vi "Trama_RMC(SubVI).vi"(0 "TRAMA":string) -> (1 "Fecha":T3, 2 "output cluster":T1, 3 "Hora":T2, 4 "Cluster":T4)   [LabVIEW 2020]
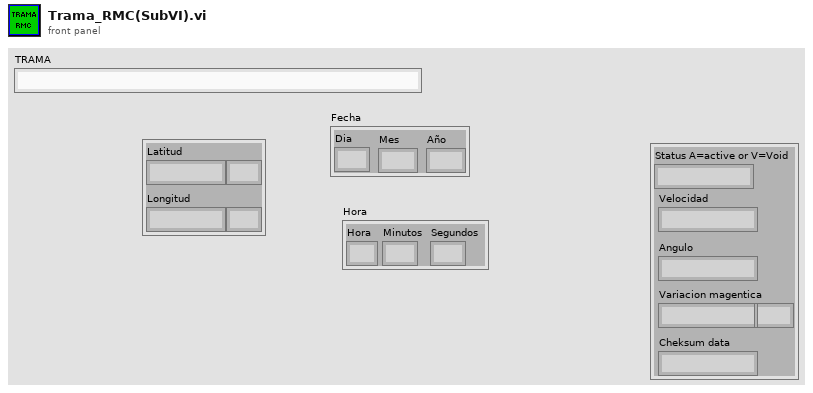
[diagram p1: front panel]
types:
  T1 = cluster{"Latitud":string, string, "Longitud":string, string}
  T2 = cluster{"Hora":string, "Segundos":string, "Minutos":string}
  T3 = cluster{"Dia":string, "Mes":string, "Año":string}
  T4 = cluster{"Status A=active or V=Void":string, "Velocidad":string, "Angulo":string, "Variacion magentica":string, string, "Cheksum data":string}
  T5 = cluster{string, string, string, string, string, string}
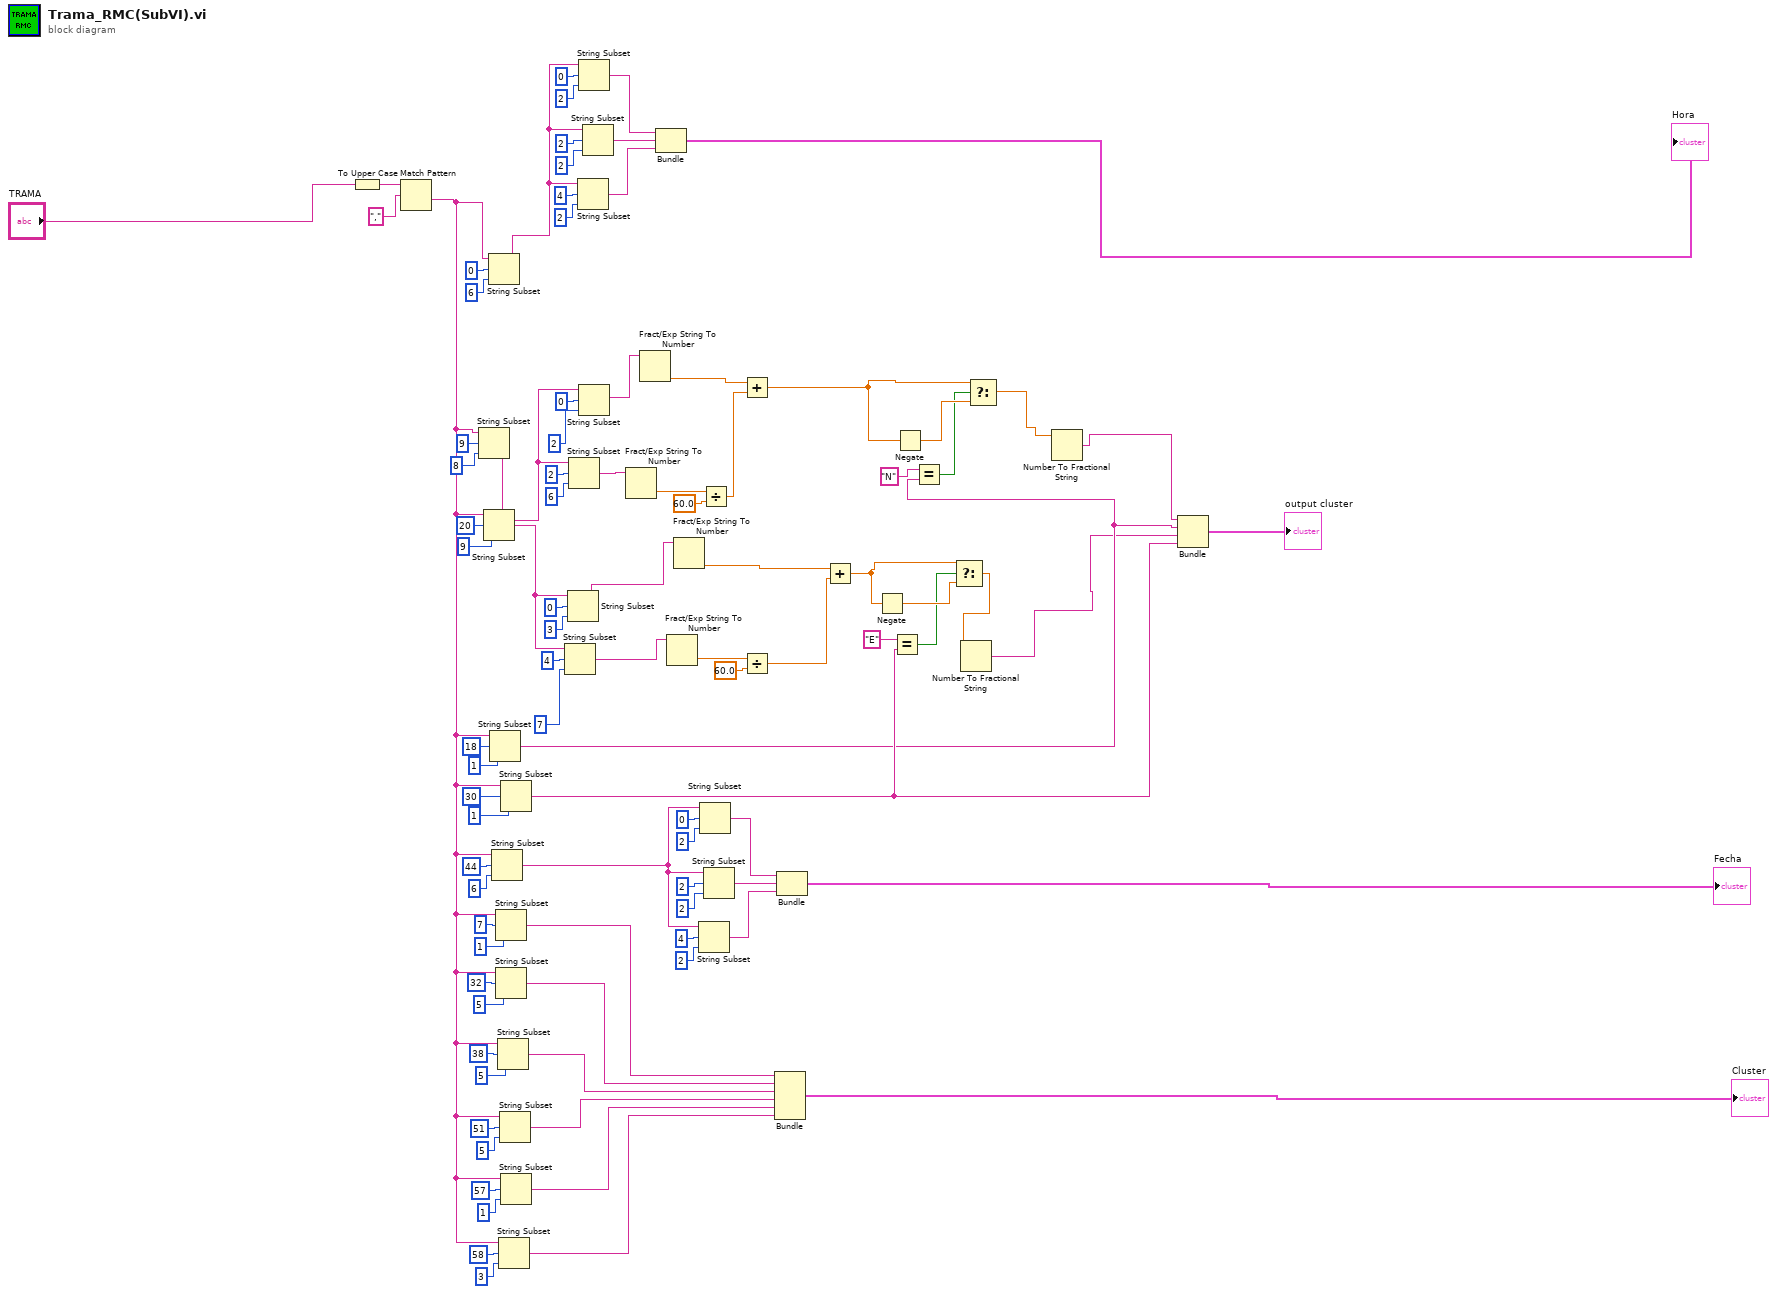
[diagram p0: block diagram]
diagram:
  n1 = To Upper Case(1:"TRAMA") -> (0:w30:string)
  n2 = Match Pattern(string=w30, regular expression=",") -> (after substring=w84:string)  [unwired: 1 in, 3 out]
  n3 = String Subset(string=w84, offset (0)=9, length (rest)=8 ("length (rest)")) -> (substring=w32:string)
  n4 = String Subset(string=w84, offset (0)=20, length (rest)=9 ("length (rest)")) -> (substring=w17:string)
  n5 = String Subset(string=w84, offset (0)=0, length (rest)=6 ("length (rest)")) -> (substring=w57:string)
  n6 = String Subset(string=w84, offset (0)=18, length (rest)=1 ("length (rest)")) -> (substring=w12:string)
  n7 = String Subset(string=w84, offset (0)=44, length (rest)=6 ("length (rest)")) -> (substring=w71:string)
  n8 = String Subset(string=w84, offset (0)=7, length (rest)=1 ("length (rest)")) -> (substring=w85:string)
  n9 = String Subset(string=w84, offset (0)=32, length (rest)=5 ("length (rest)")) -> (substring=w86:string)
  n10 = String Subset(string=w84, offset (0)=38, length (rest)=5 ("length (rest)")) -> (substring=w87:string)
  n11 = String Subset(string=w84, offset (0)=58, length (rest)=3 ("length (rest)")) -> (substring=w90:string)
  n12 = String Subset(string=w84, offset (0)=51, length (rest)=5 ("length (rest)")) -> (substring=w88:string)
  n13 = String Subset(string=w84, offset (0)=30, length (rest)=1 ("length (rest)")) -> (substring=w80:string)
  n14 = String Subset(string=w84, offset (0)=57, length (rest)=1 ("length (rest)")) -> (substring=w89:string)
  n15 = String Subset(string=w17, offset (0)=4, length (rest)=7 ("length (rest)")) -> (substring=w25:string)
  n16 = String Subset(string=w17, offset (0)=0, length (rest)=3 ("length (rest)")) -> (substring=w20:string)
  n17 = String Subset(string=w32, offset (0)=2, length (rest)=6 ("length (rest)")) -> (substring=w45:string)
  n18 = String Subset(string=w57, offset (0)=4, length (rest)=2 ("length (rest)")) -> (substring=w33:string)
  n19 = String Subset(string=w57, offset (0)=0, length (rest)=2 ("length (rest)")) -> (substring=w35:string)
  n20 = String Subset(string=w32, offset (0)=0, length (rest)=2 ("length (rest)")) -> (substring=w42:string)
  n21 = String Subset(string=w57, offset (0)=2, length (rest)=2 ("length (rest)")) -> (substring=w34:string)
  n22 = Fract/Exp String To Number(string=w45) -> (number=w44:dbl)  [unwired: 3 in, 1 out]
  n23 = Fract/Exp String To Number(string=w42) -> (number=w40:dbl)  [unwired: 3 in, 1 out]
  n24 = Bundle(w35, w34, w33) -> (→"Hora":cluster{string, string, string})  [unwired: 1 in]
  n25 = Fract/Exp String To Number(string=w25) -> (number=w24:dbl)  [unwired: 3 in, 1 out]
  n26 = Fract/Exp String To Number(string=w20) -> (number=w21:dbl)  [unwired: 3 in, 1 out]
  n27 = String Subset(string=w71, offset (0)=4, length (rest)=2 ("length (rest)")) -> (substring=w60:string)
  n28 = String Subset(string=w71, offset (0)=0, length (rest)=2 ("length (rest)")) -> (substring=w62:string)
  n29 = Divide(x=w44, y=60.0) -> (x/y=w41:dbl)
  n30 = String Subset(string=w71, offset (0)=2, length (rest)=2 ("length (rest)")) -> (substring=w61:string)
  n31 = Add(x=w40, y=w41) -> (x+y=w14:dbl)
  n32 = Divide(x=w24, y=60.0) -> (x/y=w22:dbl)
  n33 = Bundle(w85, w86, w87, w88, w89, w90) -> (→"Cluster":T5)  [unwired: 1 in]
  n34 = Bundle(w62, w61, w60) -> (→"Fecha":cluster{string, string, string})  [unwired: 1 in]
  n35 = Add(x=w21, y=w22) -> (x+y=w7:dbl)
  n36 = Negate(x=w7) -> (-x=w79:dbl)
  n37 = Equal?(x="E", y=w80) -> (x = y?=w9:bool)
  n38 = Negate(x=w14) -> (-x=w13:dbl)
  n39 = Equal?(x="N", y=w12) -> (x = y?=w10:bool)
  n40 = Select(t=w7, s=w9, f=w79) -> (s? t:f=w5:dbl)
  n41 = Number To Fractional String(number=w5) -> (F-format string=w4:string)  [unwired: 3 in]
  n42 = Select(t=w14, s=w10, f=w13) -> (s? t:f=w2:dbl)
  n43 = Number To Fractional String(number=w2) -> (F-format string=w1:string)  [unwired: 3 in]
  n44 = Bundle(w1, w12, w4, w80) -> (→"output cluster":cluster{string, string, string, string})  [unwired: 1 in]
